vi "VI Tester JUnitXML Example.vi"() -> ()   [LabVIEW 2011]
uses:
  TextTestRunner.Ant/TextTestRunner.JUnitXML.lvclass
  <vilib>/Utility/sysdir.llb/System Directory Type.ctl
  <vilib>/addons/_JKI Toolkits/VI Tester/VI Tester API.llb/Run Tests (Path).vi
  <vilib>/addons/_JKI Toolkits/VI Tester/VI Tester API.llb/VI Tester API.lvlib
panel:
  out "JUnit XML report":string
  in  "Test Path":path=path "C:/Program Files/National Instruments/LabVIEW 2009/examples/JKI/VI Tester/Queue TestCase/Queue TestCase.lvclass"
  out "error out":errorcluster
  out "test details":string
  out "successful?":bool
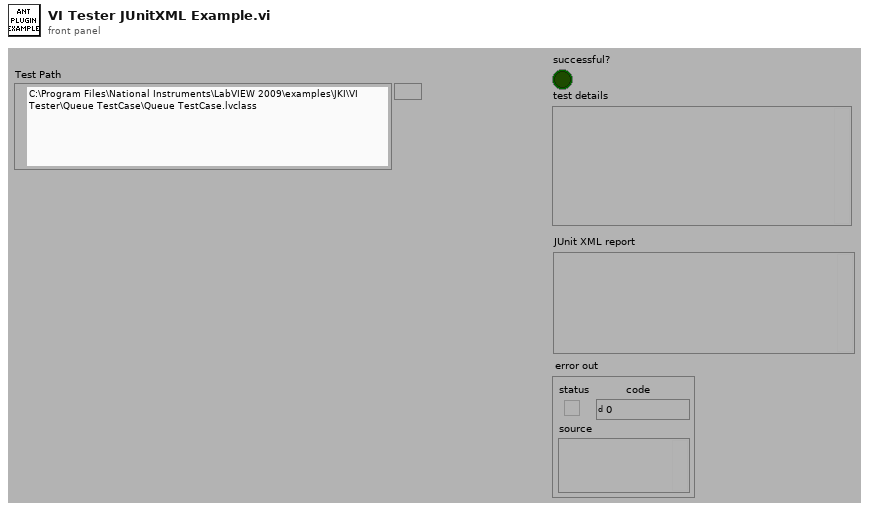
[diagram p1: front panel]
types:
  T1 = typedef "System Directory Type.ctl" = i32
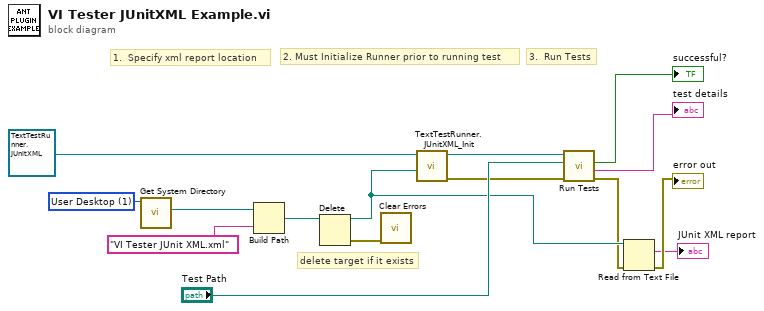
[diagram p0: block diagram]
diagram:
  w14 = T1 1 items=["User Home", "User Desktop", "User Documents", "User Application Data", "User Preferences", "User Temporary", "Public Documents", "Public Application Data", "Public Preferences", "System Core Libraries", "System Installed Libraries", "Application Files", "Boot Volume Root"] ("system directory type")
  # "3.  Run Tests"
  # "delete target if it exists"
  # "2. Must Initialize Runner prior to running test"
  # "1.  Specify xml report location"
  n1 = call <vilib>:"Get System Directory.vi"("system directory type"=w14) -> ("system directory"=w13:path)  [unwired: 10 in]
  n2 = Build Path(base path=w13, name or relative path="VI Tester JUnit XML.xml") -> (appended path=w6:path)
  n3 = Delete(path (use dialog)=w6) -> (deleted path=w4:path, error out=w5:errorcluster)  [unwired: 4 in, 1 out]
  n4 = call <vilib>:"Clear Errors.vi"("error in (no error)"=w5) -> ()  [unwired: 6 in, 1 out]
  n5 = call "TextTestRunner.JUnitXML_Init.vi"("Report Path"=w4, "TextTestRunner in"=refnum<class "TextTestRunner.JUnitXML.lvclass"> refnum ("TextTestRunner.Ant.lvclass")) -> ("error out"=w7:errorcluster, "TextTestRunner out"=w8:refnum<class "TextTestRunner.JUnitXML.lvclass">)  [unwired: 8 in]
  n6 = call-poly <vilib>:"Run Tests.vi"("TextTestRunner in"=w8, "error in (no error)"=w7, "Test Path"="Test Path") -> ("error out"=w3:errorcluster, "test details"=→"test details":string, "successful?"=→"successful?":bool)  [unwired: 6 in]
  n7 = Read from Text File(file (use dialog)=w4, error in=w3) -> (text=→"JUnit XML report":string, error out=→"error out":errorcluster)  [unwired: 2 in, 2 out]
